vi "MICSD Do RSSI.vi"(6 "Execute on Remote?(F)":bool, 7 "Use Averaging?(T)":bool=TRUE, 8 "error in (no error)":errorcluster, 9 "Measurement Type":T1(ring), 10 "Channel":u8 format="%02x", 11 "VISA Resource Name":refnum<visa-resource-name>) -> (0 "error out":errorcluster, 2 "RSSI":u16, 3 "dup VISA Resource Name":refnum<visa-resource-name>)   [LabVIEW 2020]
uses:
  <vilib>/Instr/_visa.llb/VISA Configure Serial Port (Instr).vi
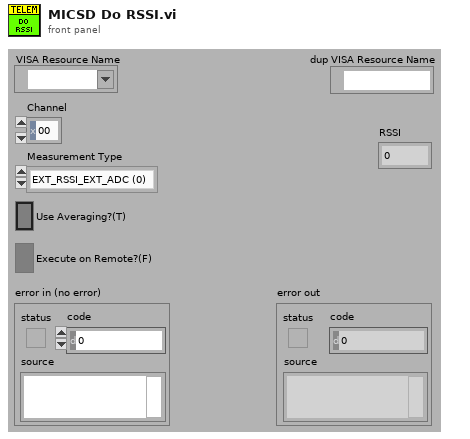
[diagram p1: front panel]
types:
  T1 = enum8{"EXT_RSSI_EXT_ADC (0)", "EXT_RSSI_INT_ADC (1)", "INT_RSSI_INT_ADC (2)"}
  T2 = cluster{"Command Token":u8, "Length":u16, "Pack Data":u8[]}
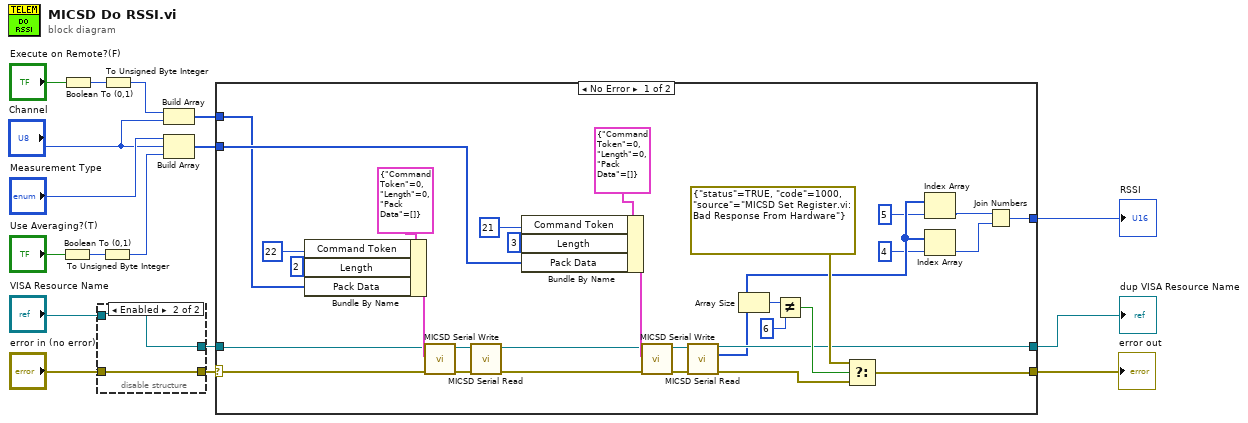
[diagram p0: block diagram]
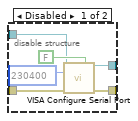
[diagram p2: hidden frame]
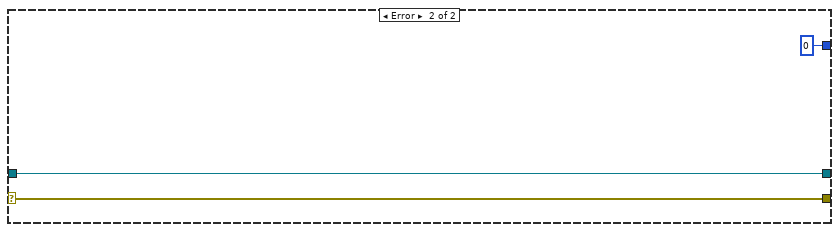
[diagram p3: hidden frame]
diagram:
  n1 = Boolean To (0,1)(Boolean="Use Averaging?(T)") -> (0, 1=w11:i16)
  n2 = Boolean To (0,1)(Boolean="Execute on Remote?(F)") -> (0, 1=w7:i16)
  n3 = disable-structure shown="Enabled" {
    disable-tunnel: [w21 w24] -> w16
    disable-tunnel: "error in (no error)" -> [w20 w24]
    disable-tunnel: "VISA Resource Name" -> [w19 w25]
    disable-tunnel: [w18 w25] -> w13
    frame Disabled {
      n4 = call-poly "VISA Configure Serial Port"("VISA resource name"=w19, "Enable Termination\nChar (T)"=FALSE ("Enable Termination\nChar (T)"), "baud rate (9600)"=u32 230400, "error in (no error)"=w20) -> ("VISA resource name out"=w18:refnum<visa-resource-name>, "error out"=w21:errorcluster)  [unwired: 10 in]
    }
    frame Enabled {
    }
  }
  n5 = To Unsigned Byte Integer(number=w11) -> (unsigned 8bit integer=w9:u8)
  n6 = To Unsigned Byte Integer(number=w7) -> (unsigned 8bit integer=w5:u8)
  n7 = Build Array(w5, "Channel") -> (w4:u8[])
  n8 = Build Array("Measurement Type", "Channel", w9) -> (w8:u8[])
  n9 = case shown="No Error" w16 {
    selector: w16 -> [w35 w59]
    tunnel: [w44 w59] -> w12
    tunnel: w13 -> [w36 w58]
    tunnel: [w46 w58] -> w17
    tunnel: w8 -> [w43 _]
    tunnel: w4 -> [w32 _]
    tunnel: [w26 u16 0] -> w3
    frame No Error {
      n10 = Bundle By Name(cluster=T2 {"Command Token"=0, "Length"=0, "Pack Data"=[]} ("Write Data"), "Command Token"=u16 22 ("Length"), "Length"=u16 2, "Pack Data"=w32) -> (w42:T2)
      n11 = call "MICSD Serial Write.vi"("error in (no error)"=w35, "Write Data"=w42, "VISA Resource Name"=w36) -> ("error out"=w38:errorcluster, "DUP Visa Resource Name"=w39:refnum<visa-resource-name>)  [unwired: 7 in]
      n12 = call "MICSD Serial Read.vi"("error in (no error)"=w38, "VISA Resource Name"=w39) -> ("error out"=w33:errorcluster, "DUP Visa Resource Name"=w34:refnum<visa-resource-name>)  [unwired: 7 in, 1 out]
      n13 = Bundle By Name(cluster=T2 {"Command Token"=0, "Length"=0, "Pack Data"=[]} ("Write Data"), "Command Token"=u16 21 ("Length"), "Length"=u16 3, "Pack Data"=w43) -> (w56:T2)
      n14 = call "MICSD Serial Write.vi"("error in (no error)"=w33, "Write Data"=w56, "VISA Resource Name"=w34) -> ("error out"=w52:errorcluster, "DUP Visa Resource Name"=w53:refnum<visa-resource-name>)  [unwired: 7 in]
      n15 = call "MICSD Serial Read.vi"("error in (no error)"=w52, "VISA Resource Name"=w53) -> ("error out"=w45:errorcluster, "Read Data"=w31:u8[], "DUP Visa Resource Name"=w46:refnum<visa-resource-name>)  [unwired: 7 in]
      n16 = Array Size(array=w31) -> (size(s)=w49:i32)
      n17 = Not Equal?(x=w49, y=6) -> (x != y?=w48:bool)
      n18 = Select(t=errorcluster {"status"=TRUE, "code"=1000, "source"="MICSD Set Register.vi:  Bad Response From Hardware"} ("error IO"), s=w48, f=w45) -> (s? t:f=w44:errorcluster)
      n19 = Index Array(array=w31, index=5) -> (element=w28:u8)
      n20 = Index Array(array=w31, index=4) -> (element=w27:u8)
      n21 = Join Numbers(hi=w28, lo=w27) -> ((hi.lo)=w26:u16)
    }
    frame Error {
    }
  }
  "dup VISA Resource Name" <- w17
  "error out" <- w12
  "RSSI" <- w3
